vi "Initialization_UserEvents.vi"(8 "error in (no error)":errorcluster, 11 "References":T2) -> (0 "error out":errorcluster, 3 "Events":refnum<event-registration>, 5 "User events":T1)   [LabVIEW 2021]
uses:
  <resource>/plugins/NIIconEditor/Controls/References Cluster.ctl
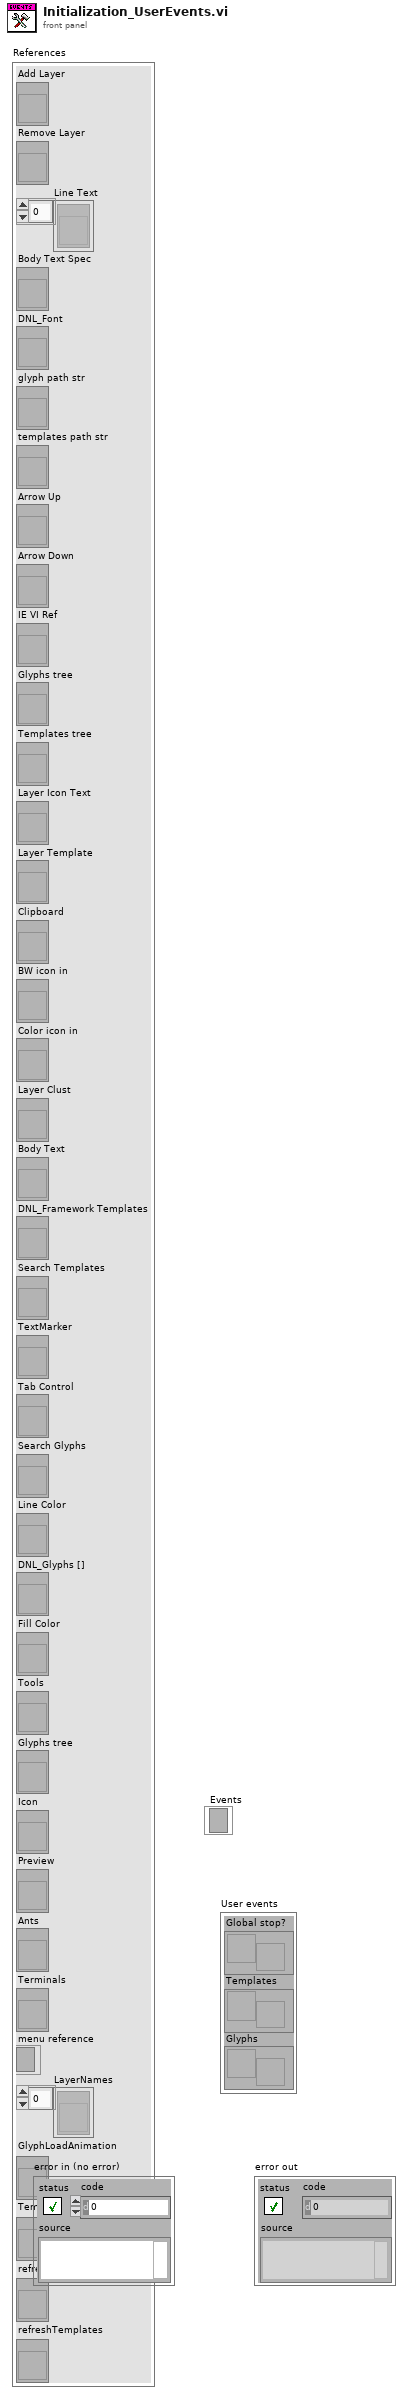
[diagram p1: front panel]
types:
  T1 = cluster{"Global stop?":refnum<user-event>, "Templates":refnum<user-event>, "Glyphs":refnum<user-event>}
  T2 = typedef "References Cluster.ctl" = cluster{"Add Layer":refnum<vi>, "Remove Layer":refnum<vi>, "Line Text":refnum<vi>[], "Body Text Spec":refnum<vi>, "DNL_Font":refnum<vi>, "glyph path str":refnum<vi>, "templates path str":refnum<vi>, "Arrow Up":refnum<vi>, "Arrow Down":refnum<vi>, "IE VI Ref":refnum<vi>, "Glyphs tree":refnum<vi>, "Templates tree":refnum<vi>, "Layer Icon Text":refnum<vi>, "Layer Template":refnum<vi>, "Clipboard":refnum<vi>, "BW icon in":refnum<vi>, "Color icon in":refnum<vi>, "Layer Clust":refnum<vi>, "Body Text":refnum<vi>, "DNL_Framework Templates":refnum<vi>, "Search Templates":refnum<vi>, "TextMarker":refnum<vi>, "Tab Control":refnum<vi>, "Search Glyphs":refnum<vi>, "Line Color":refnum<vi>, "DNL_Glyphs []":refnum<vi>, "Fill Color":refnum<vi>, "Tools":refnum<vi>, "Glyphs tree":refnum<vi>, "Icon":refnum<vi>, "Preview":refnum<vi>, "Ants":refnum<vi>, "Terminals":refnum<vi>, "menu reference":refnum<k9>, "LayerNames":refnum<vi>[], "GlyphLoadAnimation":refnum<vi>, "TemplateLoadAnimation":refnum<vi>, "refreshGlyphs":refnum<vi>, "refreshTemplates":refnum<vi>}
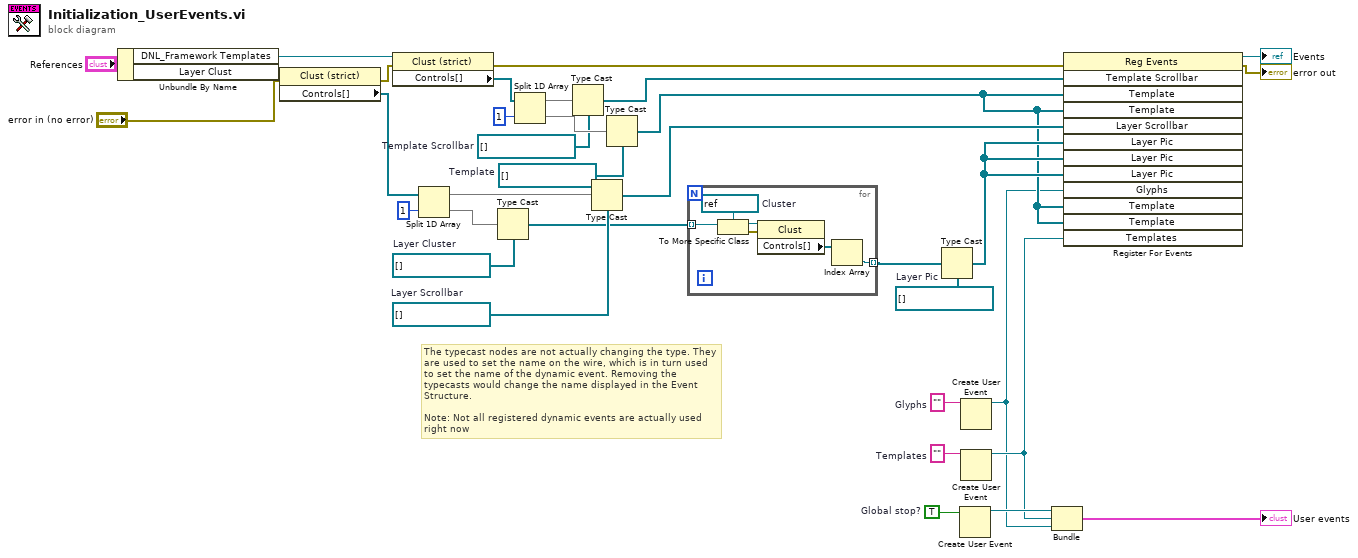
[diagram p0: block diagram]
diagram:
  w5 = TRUE  # Global stop?
  w7 = refnum<vi>[] []  # Template Scrollbar
  w8 = ""  # Templates
  w12 = refnum<vi>[] []  # Layer Pic
  w15 = refnum<vi>[] []  # Layer Scrollbar
  w17 = refnum<vi>[] []  # Template
  w21 = refnum<vi>[] []  # Layer Cluster
  w28 = ""  # Glyphs
  # "The typecast nodes are not actually changing the type. They are used to set the name on the wire, which is in turn used to set the name of the dynamic event. Removing the typecasts would change the name displayed in the Event Structure.\n\nNote: Not all registered dynamic events are actually used\nright now"
  n1 = Unbundle By Name("References") -> ("DNL_Framework Templates"=w32:refnum<vi>, "Layer Clust"=w27:refnum<vi>)
  n2 = property class="Clust (strict)"(reference=w27, error in="error in (no error)") -> (error out=w24:errorcluster, "Controls[]"=w26:refnum<vi>[])  [unwired: 1 out]
  n3 = property class="Clust (strict)"(reference=w32, error in=w24) -> (error out=w34:errorcluster, "Controls[]"=w31:refnum<vi>[])  [unwired: 1 out]
  n4 = Split 1D Array(array=w26, index=1) -> (first subarray=w16:refnum<vi>[], second subarray=w22:refnum<vi>[])
  n5 = Type Cast(type=w21, x=w22) -> (*(type *) &x=w13:refnum<vi>[])
  n6 = Split 1D Array(array=w31, index=1) -> (first subarray=w19:refnum<vi>[], second subarray=w20:refnum<vi>[])
  n7 = Type Cast(type=w7, x=w19) -> (*(type *) &x=w18:refnum<vi>[])
  n8 = Type Cast(type=w15, x=w16) -> (*(type *) &x=w14:refnum<vi>[])
  n9 = Type Cast(type=w17, x=w20) -> (*(type *) &x=w9:refnum<vi>[])
  n10 = for {
    tunnel: w13 -> [w40] mode=indexing
    tunnel: [w35] -> w11 mode=indexing
    w39 = refnum<vi> refnum  # Cluster
    n11 = To More Specific Class(target class=w39, reference=w40) -> (specific class reference=w37:refnum<vi>, error out=w38:errorcluster)  [unwired: 1 in]
    n12 = property class="Clust"(reference=w37, error in=w38) -> ("Controls[]"=w36:refnum<vi>[])  [unwired: 2 out]
    n13 = Index Array(array=w36) -> (element=w35:refnum<vi>)  [unwired: 1 in]
  }
  n14 = Type Cast(type=w12, x=w11) -> (*(type *) &x=w10:refnum<vi>[])
  n15 = Create User Event(user event datatype=w5) -> (user event=w4:refnum<user-event>)  [unwired: 1 in, 1 out]
  n16 = Create User Event(user event datatype=w28) -> (user event=w2:refnum<user-event>)  [unwired: 1 in, 1 out]
  n17 = Create User Event(user event datatype=w8) -> (user event=w3:refnum<user-event>)  [unwired: 1 in, 1 out]
  n18 = Bundle("Global stop?"=w4, "Templates"=w3, "Glyphs"=w2) -> (→"User events":T1)  [unwired: 1 out]
  n19 = register-events(error in=w34, w18, w9, w9, w14, w10, w10, w10, w2, w9, w9, w3) -> (reference out=→"Events":refnum<event-registration>, error out=→"error out":errorcluster)  [unwired: 1 in]
